vi "Set Table Colors.vi"(8 "error in (no error)":errorcluster, 11 "Controls Table Ref":refnum<vi>) -> (0 "error out":errorcluster)   [LabVIEW 2023, in "VI Properties Editor.lvlib"]
doc: "Sets the Controls table's colors based on which columns are currently editable."
uses:
  VI Properties Editor.lvlib
  <vilib>/Utility/miscctls.llb/LVRowAndColumnTypeDef.ctl
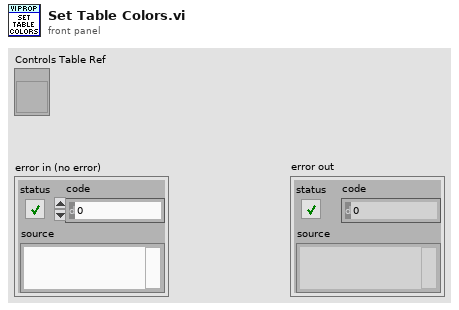
[diagram p1: front panel]
types:
  T1 = typedef "LVRowAndColumnTypeDef.ctl" = cluster{"Row":i32, "Column":i32}
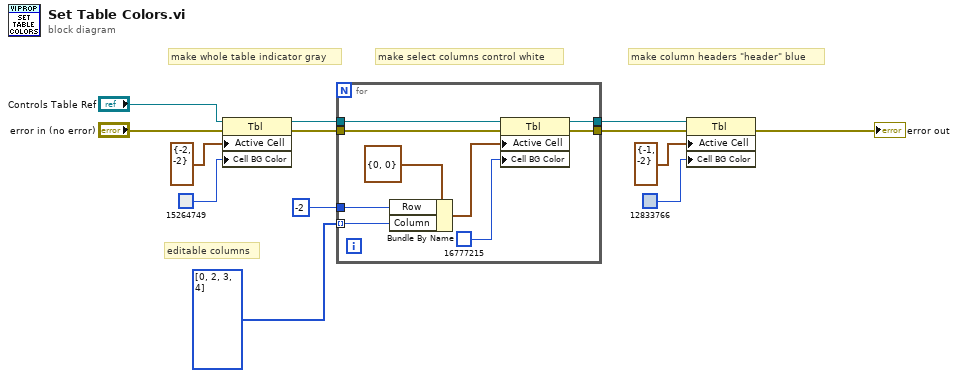
[diagram p0: block diagram]
diagram:
  # "make column headers \"header\" blue"
  # "make select columns control white"
  # "make whole table indicator gray"
  # "editable columns"
  n1 = property class="Tbl"(reference="Controls Table Ref", error in="error in (no error)", "Active Cell"=T1 {"Row"=-2, "Column"=-2} ("Active Cell:Active Cell"), "Cell BG Color"=u32 15264749 ("Active Cell:Cell Background Color")) -> (reference out=w7:refnum<vi>, error out=w6:errorcluster)
  n2 = for {
    tunnel: w7 -> [w22]
    tunnel: w6 -> [w21]
    tunnel: -2 ("Row") -> [w19]
    tunnel: i32[] [0, 2, 3, 4] -> [w18] mode=indexing
    tunnel: [w15] -> w3
    tunnel: [w14] -> w2
    n3 = Bundle By Name(cluster=T1 {"Row"=0, "Column"=0} ("Active Cell:Active Cell"), "Row"=w19, "Column"=w18) -> (w17:T1)
    n4 = property class="Tbl"(reference=w22, error in=w21, "Active Cell"=w17, "Cell BG Color"=u32 16777215 ("Active Cell:Cell Background Color")) -> (reference out=w14:refnum<vi>, error out=w15:errorcluster)
  }
  n5 = property class="Tbl"(reference=w2, error in=w3, "Active Cell"=T1 {"Row"=-1, "Column"=-2} ("Active Cell:Active Cell"), "Cell BG Color"=u32 12833766 ("Active Cell:Cell Background Color")) -> (error out=→"error out":errorcluster)  [unwired: 1 out]
